vi "DSO1K Acquire Waveform Continuously.vi"() -> ()   [LabVIEW 2009]
doc: "<B>This example shows how to use autosetup and acquire a waveform continuously on a single channel.\n\nNote: In this example, each record is acquired independently and not as a continuous stream of data.</B>"
uses:
  <instrlib>/DSO1K/Public/Data/Read Waveform (Single).vi
  <instrlib>/DSO1K/DSO1K.lvlib
panel:
  in  "Timeout (40000 ms)":u32=40000
  in  "Channel (1: Channel 1)":u16(ring)=1 items=["Channel 1"=1, "Channel 2"=2, "Channel 3"=3, "Channel 4"=4]
  out "Run Times":i32
  in  "stop":bool
  out "Waveform Graph":T1(graph)
  in  "VISA resource name":refnum<visa-resource-name>
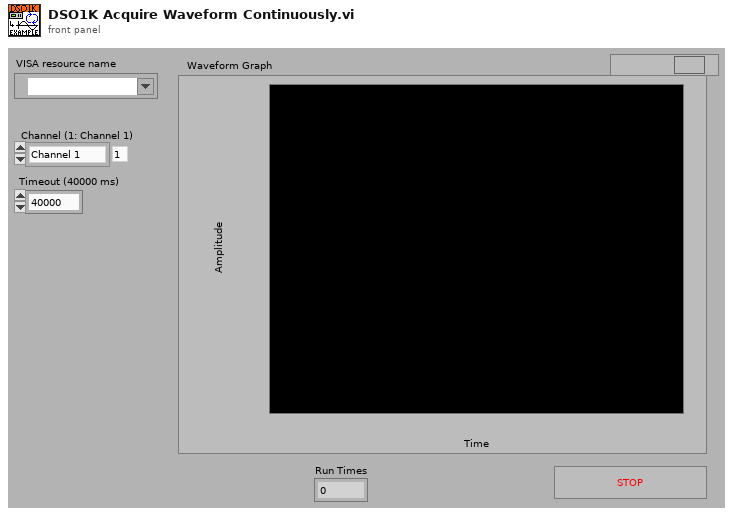
[diagram p1: front panel]
types:
  T1 = cluster{"The start time of the waveform":dbl, dbl, "Waveform":dbl[]}
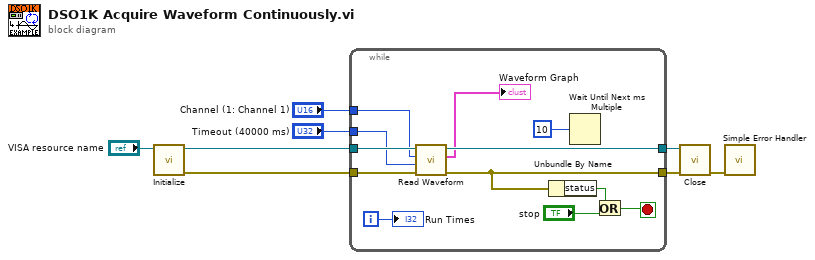
[diagram p0: block diagram]
diagram:
  n1 = call <instrlib>:"Initialize.vi"("VISA resource name"="VISA resource name") -> ("error out"=w3:errorcluster, "VISA resource name out"=w4:refnum<visa-resource-name>)  [unwired: 9 in]
  n2 = while {
    tunnel: w4 -> [w17]
    tunnel: w3 -> [w16]
    tunnel: [w20] -> w7
    tunnel: [w15] -> w6
    tunnel: "Channel (1: Channel 1)" -> [w10]
    tunnel: "Timeout (40000 ms)" -> [w9]
    i -> [w19]
    stop <- w14 stop-if-true
    n3 = call-poly <instrlib>:"Read Waveform.vi"("error in (no error)"=w16, "Timeout (40000 ms)"=w9, "Channel (1: Channel 1)"=w10, "VISA resource name"=w17) -> ("error out"=w15:errorcluster, "Waveform Graph"=→"Waveform Graph":cluster{dbl, "Sampling Period":dbl, dbl[]}, "VISA resource name out"=w20:refnum<visa-resource-name>)  [unwired: 4 in, 1 out]
    n4 = Unbundle By Name(w15) -> ("status"=w13:bool)
    n5 = Wait Until Next ms Multiple(millisecond multiple=u32 10) -> ()  [unwired: 1 out]
    n6 = Or(x=w13, y="stop") -> (x .or. y?=w14:bool)
    "Run Times" <- w19
  }
  n7 = call <instrlib>:"Close.vi"("error in (no error)"=w6, "VISA resource name"=w7) -> ("error out"=w8:errorcluster)  [unwired: 9 in]
  n8 = call <vilib>:"Simple Error Handler.vi"("error in (no error)"=w8) -> ()  [unwired: 4 in, 5 out]
